vi "Buffer for lossless tracking.vi"(5 "Ref Cluster":T2, 7 "User events":T1, 8 "error in (no error)":errorcluster, 11 "Buffer":refnum<queue>) -> (0 "error out":errorcluster)   [LabVIEW 2021]
uses:
  Controls/References Cluster.ctl
  <vilib>/Utility/miscctls.llb/LVPoint32TypeDef.ctl
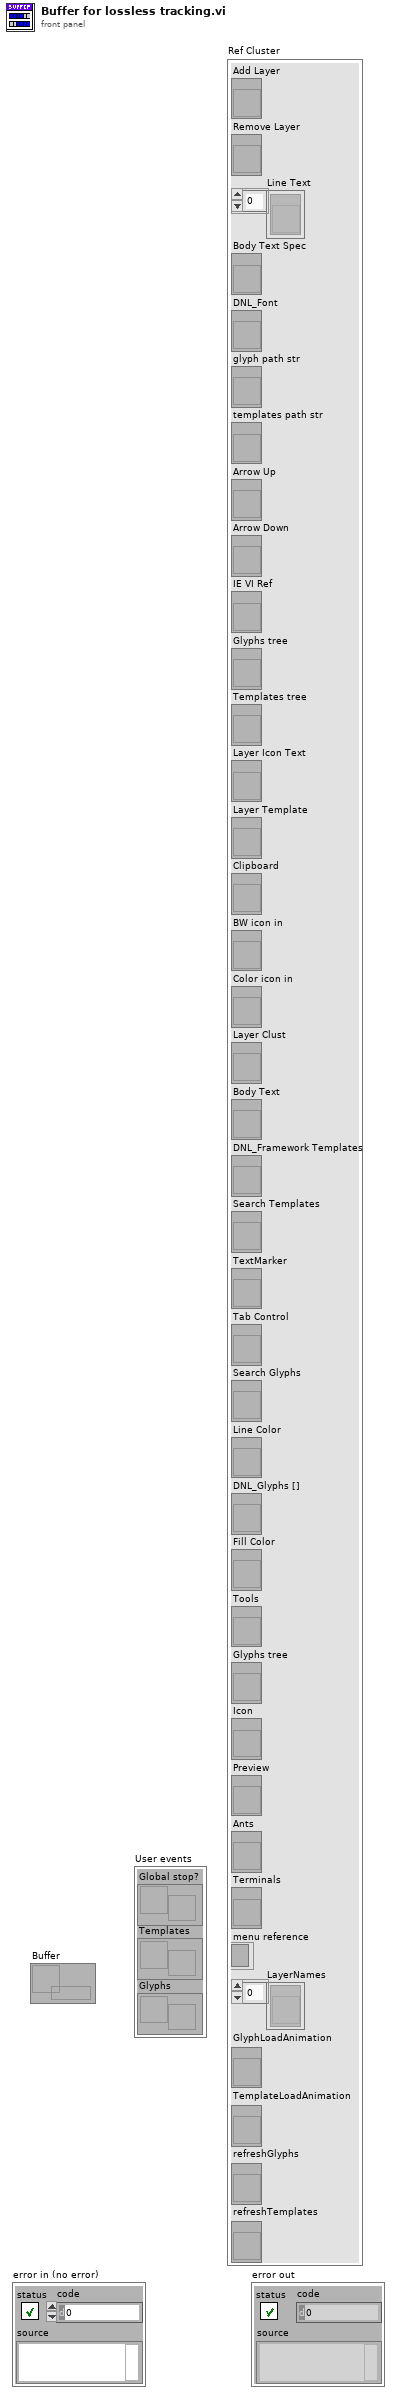
[diagram p1: front panel]
types:
  T1 = cluster{"Global stop?":refnum<user-event>, "Templates":refnum<user-event>, "Glyphs":refnum<user-event>}
  T2 = typedef "References Cluster.ctl" = cluster{"Add Layer":refnum<vi>, "Remove Layer":refnum<vi>, "Line Text":refnum<vi>[], "Body Text Spec":refnum<vi>, "DNL_Font":refnum<vi>, "glyph path str":refnum<vi>, "templates path str":refnum<vi>, "Arrow Up":refnum<vi>, "Arrow Down":refnum<vi>, "IE VI Ref":refnum<vi>, "Glyphs tree":refnum<vi>, "Templates tree":refnum<vi>, "Layer Icon Text":refnum<vi>, "Layer Template":refnum<vi>, "Clipboard":refnum<vi>, "BW icon in":refnum<vi>, "Color icon in":refnum<vi>, "Layer Clust":refnum<vi>, "Body Text":refnum<vi>, "DNL_Framework Templates":refnum<vi>, "Search Templates":refnum<vi>, "TextMarker":refnum<vi>, "Tab Control":refnum<vi>, "Search Glyphs":refnum<vi>, "Line Color":refnum<vi>, "DNL_Glyphs []":refnum<vi>, "Fill Color":refnum<vi>, "Tools":refnum<vi>, "Glyphs tree":refnum<vi>, "Icon":refnum<vi>, "Preview":refnum<vi>, "Ants":refnum<vi>, "Terminals":refnum<vi>, "menu reference":refnum<k9>, "LayerNames":refnum<vi>[], "GlyphLoadAnimation":refnum<vi>, "TemplateLoadAnimation":refnum<vi>, "refreshGlyphs":refnum<vi>, "refreshTemplates":refnum<vi>}
  T3 = typedef "LVPoint32TypeDef.ctl" = cluster{"Horizontal":i32, "Vertical":i32}
  T4 = enum32{"Pencil", "Line", "Dropper", "Fill", "Rectangle", "Filled Rectangle", "Ellipse", "Filled Ellipse", "Eraser", "Text", "Select", "Move"}
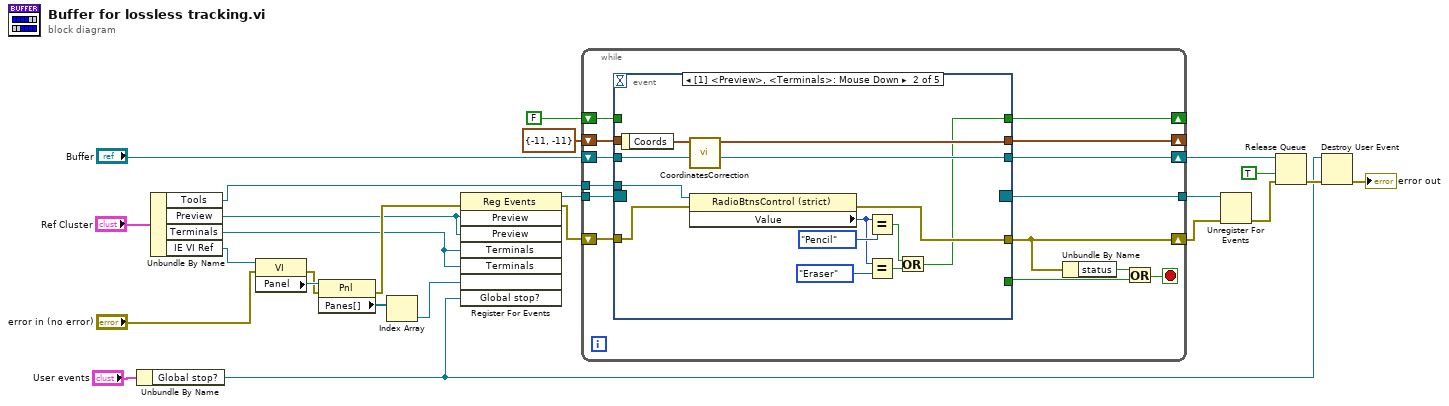
[diagram p0: block diagram]
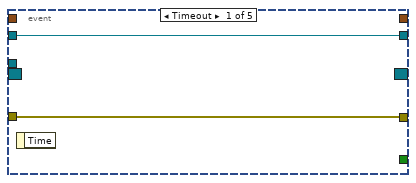
[diagram p2: hidden frame]
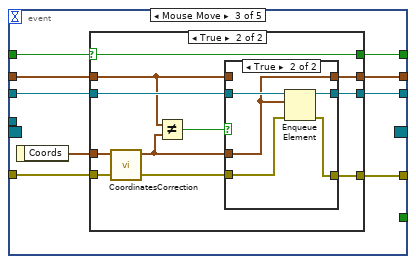
[diagram p3: hidden frame]
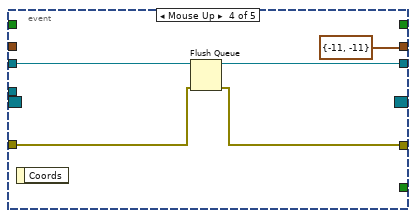
[diagram p6: hidden frame]
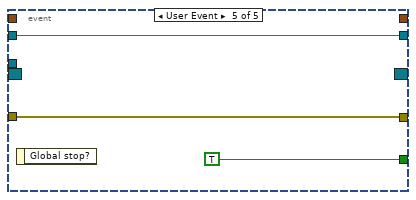
[diagram p7: hidden frame]
diagram:
  n1 = Unbundle By Name("User events") -> ("Global stop?"=w4:refnum<user-event>)
  n2 = Unbundle By Name("Ref Cluster") -> ("Tools"=w3:refnum<vi>, "Preview"=w16:refnum<vi>, "Terminals"=w1:refnum<vi>, "IE VI Ref"=w24:refnum<vi>)
  n3 = property class="VI"(reference=w24, error in="error in (no error)") -> (error out=w22:errorcluster, "Panel"=w23:refnum<vi>)  [unwired: 1 out]
  n4 = property class="Pnl"(reference=w23, error in=w22) -> (error out=w19:errorcluster, "Panes[]"=w21:refnum<vi>[])  [unwired: 1 out]
  n5 = Index Array(array=w21) -> (element=w20:refnum<vi>)  [unwired: 1 in]
  n6 = register-events(error in=w19, w16, w16, w1, w1, w20, w4) -> (reference out=w14:refnum<event-registration>, error out=w18:errorcluster)  [unwired: 1 in]
  n7 = while {
    tunnel: w14 -> [w39]
    shift-right: [w35] -> _
    shift-left: FALSE -> [w37]
    tunnel: [w36] -> w15
    shift-right: [w33] -> w13
    shift-left: w18 -> [w38]
    shift-right: [w29] -> w11
    shift-left: "Buffer" -> [w34]
    tunnel: w3 -> [w28]
    shift-right: [w27] -> _
    shift-left: T3 {"Horizontal"=-11, "Vertical"=-11} ("Corrected Out") -> [w26]
    stop <- w30 stop-if-true
    n8 = event shown="[1] <Preview>, <Terminals>: Mouse Down" {
      selector: w39 -> [_ _ _ _ _]
      dyn-events: [_ _ _ _ _] -> w36
      timeout: _ -> [_ _ _ _ _]
      tunnel: w38 -> [w41 w51 w59 w86 w90]
      tunnel: w37 -> [_ _ w62 _ _]
      tunnel: [_ _ _ _ TRUE] -> w31
      tunnel: [_ w42 w57 _ _] -> w35
      tunnel: w34 -> [w40 w53 w61 w88 w89]
      tunnel: [w41 w52 w58 w85 w90] -> w33
      tunnel: [w40 w53 w56 w87 w89] -> w29
      tunnel: w28 -> [_ w50 _ _ _]
      tunnel: [_ w47 w54 T3 {"Horizontal"=-11, "Vertical"=-11} ("Corrected Out") _] -> w27
      tunnel: w26 -> [_ _ w55 _ _]
      event Timeout {
        n9 = event-data() -> ()  [unwired: 1 in, 1 out]
      }
      event Mouse Down {
        n10 = event-data() -> ("Coords"=w48:T3)  [unwired: 1 in]
        n11 = call "CoordinatesCorrection.vi"("Coordinates In"=w48) -> ("Corrected Out"=w47:T3)  [unwired: 10 out]
        n12 = property class="RadioBtnsControl (strict)"(reference=w50, error in=w51) -> (error out=w52:errorcluster, "Value"=w46:T4)  [unwired: 1 out]
        n13 = Equal?(x=w46, y=T4."Pencil") -> (x = y?=w43:bool)
        n14 = Equal?(x=w46, y=T4."Eraser") -> (x = y?=w44:bool)
        n15 = Or(x=w43, y=w44) -> (x .or. y?=w42:bool)
      }
      event Mouse Move {
        n16 = event-data() -> ("Coords"=w60:T3)  [unwired: 1 in]
        n17 = case shown="True" w62 {
          selector: w62 -> [_ w72]
          tunnel: w61 -> [w64 w75]
          tunnel: w60 -> [_ w70]
          tunnel: w59 -> [w65 w74]
          tunnel: [w65 w73] -> w58
          tunnel: [_ w72] -> w57
          tunnel: [w64 w71] -> w56
          tunnel: w55 -> [w63 w66]
          tunnel: [w63 w67] -> w54
          frame False {
          }
          frame True {
            n18 = call "CoordinatesCorrection.vi"("Coordinates In"=w70) -> ("Corrected Out"=w69:T3)  [unwired: 10 out]
            n19 = Not Equal?(x=w66, y=w69) -> (x != y?=w68:bool)
            n20 = case shown="True" w68 {
              tunnel: w75 -> [w77 w83]
              tunnel: w74 -> [w76 w82]
              tunnel: [w76 w81] -> w73
              tunnel: [w77 w80] -> w71
              tunnel: w69 -> [_ w79]
              tunnel: [w78 w79] -> w67
              tunnel: w66 -> [w78 _]
              frame False {
              }
              frame True {
                n21 = Enqueue Element(queue=w83, element=w79, error in (no error)=w82) -> (queue out=w80:refnum<queue>, error out=w81:errorcluster)  [unwired: 1 in, 1 out]
              }
            }
          }
        }
      }
      event Mouse Up {
        n22 = event-data() -> ()  [unwired: 1 in, 1 out]
        n23 = Flush Queue(queue=w88, error in (no error)=w86) -> (queue out=w87:refnum<queue>, error out=w85:errorcluster)  [unwired: 1 out]
      }
      event User Event {
        n24 = event-data() -> ()  [unwired: 1 in, 1 out]
      }
    }
    n25 = Unbundle By Name(w33) -> ("status"=w32:bool)
    n26 = Or(x=w32, y=w31) -> (x .or. y?=w30:bool)
  }
  n27 = Unregister For Events(event registration refnum=w15, error in=w13) -> (error out=w9:errorcluster)
  n28 = Release Queue(queue=w11, force destroy? (F)=TRUE, error in (no error)=w9) -> (error out=w8:errorcluster)  [unwired: 2 out]
  n29 = Destroy User Event(user event=w4, error in=w8) -> (error out=→"error out":errorcluster)
